vi "Low Goal Targeting.vi"(8 "Camera Address":string="axis-camera.local") -> (0 "Results":T2={"Distance (ft)"=4.321737523800672, "Error"=51.25000000000001, "Normalized"={"Center"={-0.018749999999999933, -0.08333333333333326}, "Rectangle"={"Numeric"=-0.17499999999999993, "Numeric 2"=0.033333333333333326, "Numeric 3"=0.13749999999999996, "Numeric 5"=-0.19999999999999996}}, "Pixels"={"Center"={157.0, 130.0}, "Rectangle"={"Numeric"=132.0, "Numeric 2"=116.0, "Numeric 3"=182.0, "Numeric 5"=144.0}}} {"Error" format="%#_3g"; "Pixels"."Rectangle"."Numeric 5" format="%#_3g"; "Pixels"."Rectangle"."Numeric 3" format="%#_3g"; "Pixels"."Rectangle"."Numeric 2" format="%#_3g"; "Pixels"."Rectangle"."Numeric" format="%#_3g"; "Normalized"."Rectangle"."Numeric 5" format="%#_2g"; "Normalized"."Rectangle"."Numeric 3" format="%#_2g"; "Normalized"."Rectangle"."Numeric 2" format="%#_2g"; "Normalized"."Rectangle"."Numeric" format="%#_2g"; "Normalized"."Center"."?" format="%#_3g"; "Normalized"."Center"."?" format="%#_3g"; "Distance (ft)" format="%#_3g"}, 1 "Mask":T1(plugin-control), 3 "Original Image":T1(plugin-control))   [LabVIEW 2023]
uses:
  <vilib>/vision/NI_Vision_Development_Module.lvlib
  <vilib>/vision/driver/NI_Vision_Acquisition_Software.lvlib
  Vision Cluster Type Def.ctl
panel:
  in  "error in":errorcluster
  in  "Tab Control":enum32{"Vision", "Misc"}(tab)
  out "Qualified Particles":i32=2
  out "Top Score":dbl=51.25000000000001
  out "Error":errorcluster
  out "Acquired Frames/s":dbl=29.98065764023211
  out "Processed Frames/s":dbl=12.572533849129593
  out "Missed Frames":bool=TRUE
  in  "Red or Hue Range":cluster{"Lower value":i32, "Upper value":i32}={"Lower value"=74, "Upper value"=200}
  in  "Green or Sat Range":cluster{"Lower value":i32, "Upper value":i32}={"Lower value"=250, "Upper value"=255}
  out "Center":dbl=-0.018749999999999933 format="%.6g"
  in  "Blue or Luma or Val or Inten Range":cluster{"Lower value":i32, "Upper value":i32}={"Lower value"=50, "Upper value"=200}
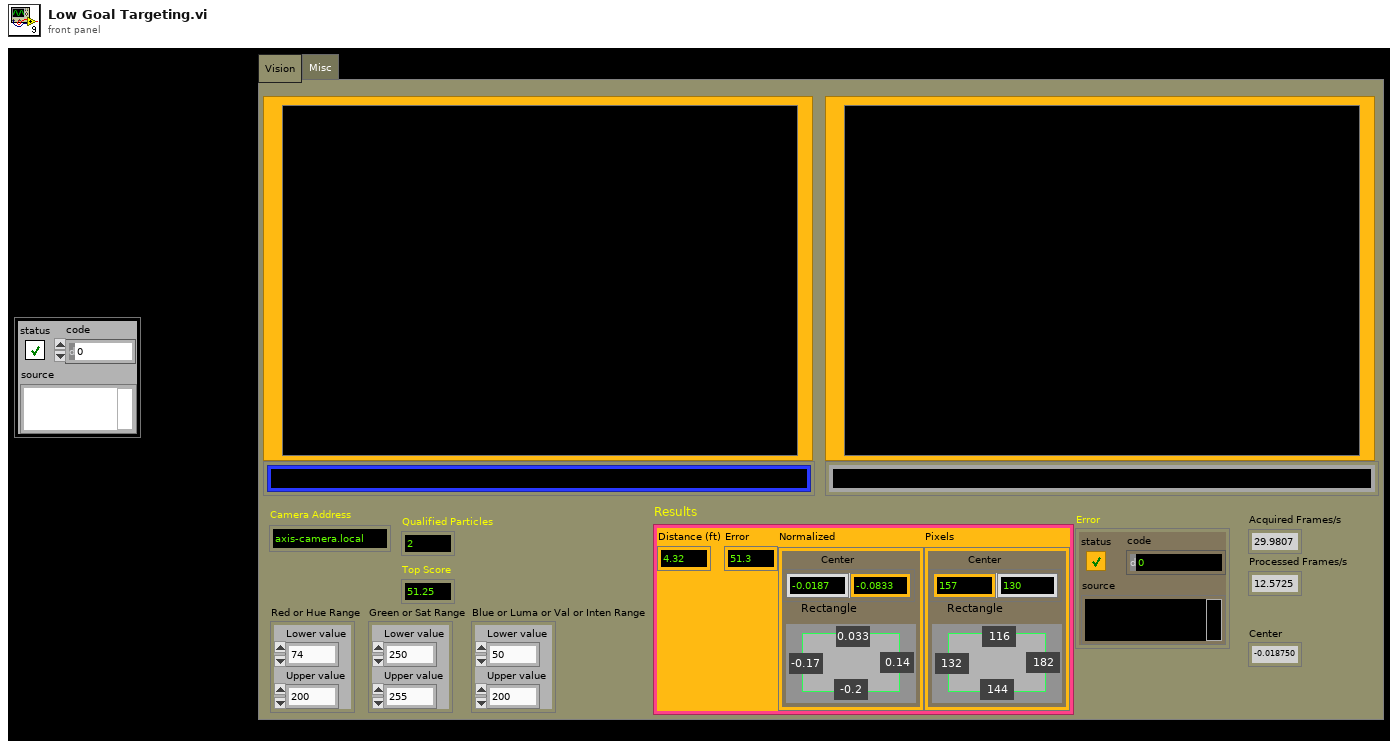
[diagram p1: front panel]
types:
  T1 = typedef "IMAQ Image.ctl" = refnum<image>
  T2 = cluster{"Distance (ft)":dbl, "Error":dbl, "Normalized":cluster{"Center":cluster{dbl, dbl}, "Rectangle":cluster{"Numeric":dbl, "Numeric 2":dbl, "Numeric 3":dbl, "Numeric 5":dbl}}, "Pixels":cluster{"Center":cluster{dbl, dbl}, "Rectangle":cluster{"Numeric":dbl, "Numeric 2":dbl, "Numeric 3":dbl, "Numeric 5":dbl}}}
  T3 = typedef "Particle Parameters" = i32
  T4 = typedef "Image Type" = u32
  T5 = typedef "IMAQdx.ctl" = refnum<k21>
  T6 = typedef "Vision Cluster Type Def.ctl" = cluster{"Distance":dbl, "Angle":dbl, "Particle":dbl, "Score":dbl, "loop time":dbl, "Communication":bool}
  T7 = cluster{"Left":dbl, "Top":dbl, "Right":dbl, "Bottom":dbl}
  T8 = cluster{"Distance (ft)":dbl, "Score":dbl, "Normalized":cluster{"Center":cluster{dbl, dbl}, "Rectangle":cluster{"Numeric":dbl, "Numeric 2":dbl, "Numeric 3":dbl, "Numeric 5":dbl}}, "Pixels":cluster{"Center":cluster{dbl, dbl}, "Rectangle":cluster{"Numeric":dbl, "Numeric 2":dbl, "Numeric 3":dbl, "Numeric 5":dbl}}}
  T9 = cluster{cluster{"Lower":dbl, "Upper":dbl}, cluster{"Lower":dbl, "Upper":dbl}, cluster{"Lower":dbl, "Upper":dbl}}
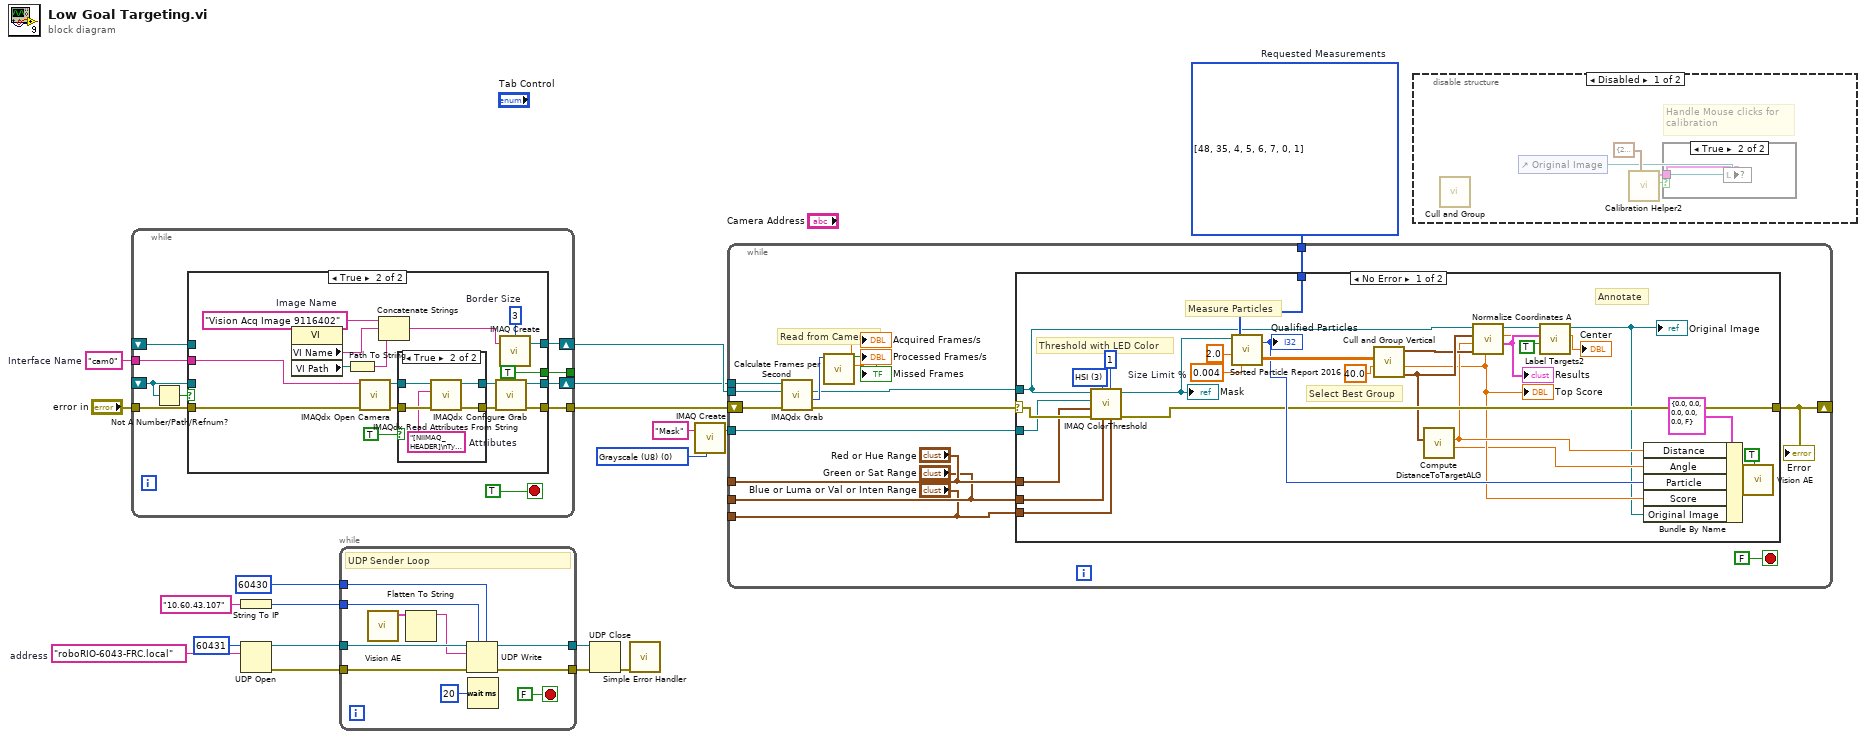
[diagram p0: block diagram]
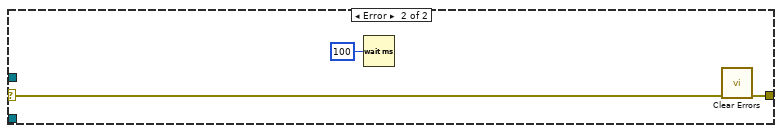
[diagram p6: hidden frame]
diagram:
  w6 = "cam0"  # Interface Name
  w2 = "roboRIO-6043-FRC.local"  # address
  w16 = T3[] [48, 35, 4, 5, 6, 7, 0, 1] items=["Center of Mass X", "Center of Mass Y", "First Pixel X", "First Pixel Y", "Bounding Rect Left", "Bounding Rect Top", "Bounding Rect Right", "Bounding Rect Bottom", "Max Feret Diameter Start X", "Max Feret Diameter Start Y", "Max Feret Diameter End X", "Max Feret Diameter End Y", "Max Horiz. Segment Length Left", "Max Horiz. Segment Length Right", "Max Horiz. Segment Length Row", "-", "Bounding Rect Width", "Bounding Rect Height", "Bounding Rect Diagonal", "Perimeter", "Convex Hull Perimeter", "Holes' Perimeter", "Max Feret Diameter", "Equivalent Ellipse Major Axis", "Equivalent Ellipse Minor Axis", "Equivalent Ellipse Minor Axis (Feret)", "Equivalent Rect Long Side", "Equivalent Rect Short Side", "Equivalent Rect Diagonal", "Equivalent Rect Short Side (Feret)", "Average Horiz. Segment Length", "Average Vert. Segment Length", "Hydraulic Radius", "Waddel Disk Diameter", "-", "Area", "Holes' Area", "Particle & Holes' Area", "Convex Hull Area", "Image Area", "-", "Number of Holes", "Number of Horiz. Segments", "Number of Vert. Segments", "-", "Orientation", "Max Feret Diameter Orientation", "-", "% Area/Image Area", "% Area/(Particle & Holes' Area)", "Ratio of Equivalent Ellipse Axes", "Ratio of Equivalent Rect Sides", "-", "Elongation Factor", "Compactness Factor", "Heywood Circularity Factor", "Type Factor", "-", "Sum X", "Sum Y", "Sum XX", "Sum XY", "Sum YY", "Sum XXX", "Sum XXY", "Sum XYY", "Sum YYY", "-", "Moment of Inertia XX", "Moment of Inertia XY", "Moment of Inertia YY", "Moment of Inertia XXX", "Moment of Inertia XXY", "Moment of Inertia XYY", "Moment of Inertia YYY", "Norm. Moment of Inertia XX", "Norm. Moment of Inertia XY", "Norm. Moment of Inertia YY", "Norm. Moment of Inertia XXX", "Norm. Moment of Inertia XXY", "Norm. Moment of Inertia XYY", "Norm. Moment of Inertia YYY", "Hu Moment 1", "Hu Moment 2", "Hu Moment 3", "Hu Moment 4", "Hu Moment 5", "Hu Moment 6", "Hu Moment 7"]  # Requested Measurements
  w19 = T4 0 items=["Grayscale (U8)", "Grayscale (I16)", "Grayscale (SGL)", "Complex (CSG)", "RGB (U32)", "HSL (U32)", "RGB (U64)", "Grayscale (U16)"] ("Image Type")
  n1 = while "While Loop_template0" {
    shift-right: [w29] -> w3
    shift-left: _ -> [w22]
    tunnel: [w28] -> w5
    tunnel: "error in" -> [w27]
    shift-right: [w25] -> w4
    shift-left: _ -> [w24]
    tunnel: w6 -> [w23]
    tunnel: [w20] -> _
    stop <- TRUE ("_template0") stop-if-true
    n2 = Not A Number/Path/Refnum?(number/path/refnum=w22) -> (NaN/Path/Refnum?=w21:bool)
    n3 = case "Case Structure_template0" shown="True" w21 {
      tunnel: [w32 w48] -> w29
      tunnel: w22 -> [w32 _]
      tunnel: [w31 w47] -> w28
      tunnel: w27 -> [w31 w49]
      tunnel: [w30 w46] -> w25
      tunnel: w24 -> [w30 _]
      tunnel: w23 -> [_ w36]
      tunnel: [_ TRUE] -> w20
      frame False {
      }
      frame True {
        w33 = 3  # Border Size
        w41 = "Vision Acq Image 9116402"  # Image Name
        n4 = property class="VI"() -> ("VI Name"=w44:string, "VI Path"=w45:path)  [unwired: 2 in, 2 out]
        n5 = Path To String(path=w45) -> (string=w43:string)
        n6 = call <vilib>:"IMAQdx Open Camera.vi"("error in"=w49, "Session In"=w36) -> ("error out"=w39:errorcluster, "Session Out"=w40:T5)  [unwired: 1 in, 7 out]
        n7 = Concatenate Strings(w41, w44, w43) -> (w42:string)
        n8 = case shown="True" TRUE ("Init Attributes") {
          tunnel: w40 -> [w51 w56]
          tunnel: w39 -> [w50 w55]
          tunnel: [w51 w53] -> w38
          tunnel: [w50 w52] -> w37
          frame False {
          }
          frame True {
            w54 = "[NIIMAQ_HEADER]\nType = 2\nVersion = 8\n\n[CAMERA_DATA]\nAcquisitionAttributes::Bayer::Algorithm = \"Bilinear\"\nAcquisitionAttributes::Bayer::GainB = \"1\"\nAcquisitionAttributes::Bayer::GainG = \"1\"\nAcquisitionAttributes::Bayer::GainR = \"1\"\nAcquisitionAttributes::Bayer::Pattern = \"Use hardware value\"\nAcquisitionAttributes::BitsPerPixel = \"Use hardware value\"\nAcquisitionAttributes::IgnoreFirstFrame = \"false\"\nAcquisitionAttributes::ImageDecoderCopyMode = \"Auto\"\nAcquisitionAttributes::OutputImageType = \"Auto\"\nAcquisitionAttributes::OverwriteMode = \"Get Newest\"\nAcquisitionAttributes::PixelSignedness = \"Use hardware value\"\nAcquisitionAttributes::ReceiveTimestampMode = \"None\"\nAcquisitionAttributes::ShiftPixelBits = \"false\"\nAcquisitionAttributes::SwapPixelBytes = \"false\"\nAcquisitionAttributes::Throttling::MaximumBandwidth = \"10000\"\nAcquisitionAttributes::Throttling::MaximumFrameRate = \"100\"\nAcquisitionAttributes::Timeout = \"5000\"\nAcquisitionAttributes::VideoMode = \"Default Camera Stream\"\nCameraAttributes::Authentication::Password = \"\"\nCameraAttributes::Authentication::UserName = \"\"\nCameraAttributes::Compression::JPEGCompressionLevel = \"30\"\nCameraAttributes::FrameRateLimit::Enabled = \"false\"\nCameraAttributes::FrameRateLimit::Value = \"30\"\nCameraAttributes::ImageControls::VerticalFlip = \"false\"\n"  # Attributes
            n9 = call <vilib>:"IMAQdx Read Attributes From String.vi"("error in"=w55, "Attributes String In"=w54, "Session In"=w56) -> ("error out"=w52:errorcluster, "Session Out"=w53:T5)  [unwired: 7 out]
          }
        }
        n10 = call <vilib>:"IMAQdx Configure Grab.vi"("error in"=w37, "Session In"=w38) -> ("error out"=w47:errorcluster, "Session Out"=w48:T5)  [unwired: 1 in, 7 out]
        n11 = call "IMAQ Create"("Border Size"=w33, "Image Name"=w42) -> ("New Image"=w46:T1)  [unwired: 2 in, 2 out]
      }
    }
  }
  n12 = String To IP(1:"10.60.43.107" ("name")) -> (0:w12:u32)
  n13 = UDP Open(10:w2, 11:u16 60431 ("port")) -> (port=w11:refnum<k16>, 0:w10:errorcluster)  [unwired: 3 in, 1 out]
  n14 = while {
    tunnel: [w63] -> w14
    tunnel: w11 -> [w66]
    tunnel: w10 -> [w65]
    tunnel: [w64] -> w15
    tunnel: w12 -> [w62]
    tunnel: u16 60430 ("remote port") -> [w60]
    stop <- FALSE stop-if-true
    # "UDP Sender Loop"
    n15 = call "Vision AE.vi"() -> ("Vision Cluster (out)"=w59:T6)  [unwired: 11 in]
    n16 = Flatten To String(anything=w59) -> (data string=w58:string)  [unwired: 3 in, 2 out]
    n17 = UDP Write(address=w62, port or service name=w60, connection ID=w66, data in=w58, 8:w65) -> (error out=w63:errorcluster, 3:w64:refnum<k16>)  [unwired: 1 in]
    n18 = Wait (ms)(milliseconds to wait=u32 20) -> ()  [unwired: 1 out]
  }
  n19 = UDP Close(connection ID=w15, 8:w14) -> (error out=w13:errorcluster)  [unwired: 1 out]
  n20 = call <vilib>:"Simple Error Handler.vi"("error in (no error)"=w13) -> ()  [unwired: 4 in, 5 out]
  n21 = call "IMAQ Create"("Image Name"="Mask", "Image Type"=w19) -> ("New Image"=w17:T1)  [unwired: 2 in, 2 out]
  n22 = while {
    tunnel: w4 -> [w77]
    tunnel: w17 -> [w81]
    tunnel: w16 -> [w80]
    tunnel: w3 -> [w78]
    shift-right: [w79] -> _
    shift-left: w5 -> [w76]
    tunnel: ["Red or Hue Range"] -> _
    tunnel: ["Green or Sat Range"] -> _
    tunnel: ["Blue or Luma or Val or Inten Range"] -> _
    stop <- FALSE stop-if-true
    # "Read from Camera"
    n23 = call <vilib>:"IMAQdx Grab.vi"("error in"=w76, "Image In"=w77, "Session In"=w78) -> ("error out"=w75:errorcluster, "Buffer Number Out"=w74:u32, "Image Out"=w70:T1)  [unwired: 1 in, 5 out]
    n24 = call <vilib>:"Calculate Frames per Second.vi"("Buffer Number"=w74) -> ("Missed Frames"=→"Missed Frames":bool, "Processed Frames/s"=→"Processed Frames/s":dbl, "Acquired Frames/s"=→"Acquired Frames/s":dbl)  [unwired: 2 in, 6 out]
    n25 = case shown="No Error" w75 {
      selector: w75 -> [w101 w112]
      tunnel: w81 -> [w95 _]
      tunnel: w80 -> [w111 _]
      tunnel: w70 -> [w87 _]
      tunnel: [w100 w113] -> w79
      tunnel: "Red or Hue Range" -> [w98 _]
      tunnel: "Green or Sat Range" -> [w97 _]
      tunnel: "Blue or Luma or Val or Inten Range" -> [w96 _]
      frame No Error {
        w102 = u16 3 items=["RGB", "HSL", "HSV", "HSI"] ("Color Mode")
        w110 = 0.004  # Size Limit %
        # "Measure Particles"
        # "Annotate"
        # "Select Best Group"
        # "Threshold with LED Color"
        n26 = call "IMAQ ColorThreshold"("Blue or Luma or Val or Inten Range"=w96, "Replace Value"=1, "Green or Sat Range"=w97, "Color Mode"=w102, "error in (no error)"=w101, "Red or Hue Range"=w98, "Image Dst"=w95, "Image Src"=w87) -> ("error out"=w100:errorcluster, "Image Dst Out"=w99:T1)  [unwired: 2 out]
        "Mask" <- w99
        n27 = call "Sorted Particle Report 2016.vi"("Min Area Size %"=w110, "Particle Count Limit"=2.0 ("Particles"), "Pixel Measurements"=w111, "Image in"=w99) -> ("Sorted Data"=w107:dbl[][], "Particles"=w105:i32)
        "Qualified Particles" <- w105
        n28 = call "Cull and Group Vertical.vi"("Score Cutoff"=40.0, "Sorted Data"=w107) -> ("Rect"=w94:T7, "Top Score"=w89:dbl, "Center"=w93:cluster{"X":dbl, "Y":dbl})  [unwired: 6 in, 1 out]
        "Top Score" <- w89
        n29 = call "Compute DistanceToTargetALG.vi"("Line"=w94) -> ("Angle to Target"=w86:dbl, "Distance (ft)"=w92:dbl)  [unwired: 8 in, 1 out]
        n30 = call "Normalize Coordinates A.vi"("Score"=w89, "Center"=w93, "Distance"=w92, "Bounding box"=w94, "Image in"=w87) -> ("Results"=w90:T8, "Center"=→"Center":dbl, "Image out"=w91:T1)  [unwired: 4 in]
        "Results" <- w90
        n31 = call "Label Targets2.vi"("Annotate"=TRUE, "Results"=w90, "Image in"=w91) -> ("Image out"=w83:T1)  [unwired: 8 in]
        "Original Image" <- w83
        n32 = Bundle By Name(cluster=T6 {"Distance"=0.0, "Angle"=0.0, "Particle"=0.0, "Score"=0.0, "loop time"=0.0, "Communication"=FALSE} ("Vision Cluster (in)"), "Distance"=w92, "Angle"=w86, "Particle"=w105, "Score"=w89, "Original Image"=w83) -> (w84:T6)
        n33 = call "Vision AE.vi"("Update"=TRUE, "Vision Cluster (in)"=w84) -> ()  [unwired: 9 in, 1 out]
      }
      frame Error {
        n34 = Wait (ms)(milliseconds to wait=u32 100) -> ()  [unwired: 1 out]
        n35 = call <vilib>:"Clear Errors.vi"("error in (no error)"=w112) -> ("error out"=w113:errorcluster)  [unwired: 5 in, 1 out]
      }
    }
    "Error" <- w79
  }
  n36 = disable-structure shown="Disabled" {
    frame Disabled {
      # "Handle Mouse clicks for\ncalibration"
      n37 = call "Cull and Group.vi"() -> ()  [unwired: 8 in, 4 out]
      n38 = control-ref of="Original Image"() -> (w115:refnum<vi>)
      n39 = call "Calibration Helper2.vi"("Std Devs"=cluster{"H":dbl, "S":dbl, "V":dbl} {"H"=2.0, "S"=6.0, "V"=6.0} ("Std Devs for Calibration"), "Image Ctl Refnum"=w115) -> ("Changed"=w116:bool, "output color"=w117:T9, 9:w118)  [unwired: 7 in]
      n40 = case shown="True" w116 {
        tunnel: w117 -> [_ w120]
        frame False {
        }
        frame True {
          n41 = local write item#-1(w120) -> ()
        }
      }
    }
    frame Enabled {
    }
  }
